vi "Stop Core.vi"(10 "final error code":i32, 11 "DAQ in":refnum<class "DAQ.lvclass">) -> (3 "DAQ out":refnum<class "DAQ.lvclass">)   [LabVIEW 2011, in "DAQ.lvclass"]
doc: "(<B>Filename</B>: Actor Framework.lvlib:Actor.lvclass:Stop Core.vi)\n\nDefines what the actor does before it stops. Use the <B>final error code</B> input to determine whether the actor shut down in response to an error.\n\nBy default, this method does nothing. A descendant class may override it to define behavior, such as shutting down any processes the actor initiated in its override of the Actor Core method."
uses:
  DAQ.lvclass
  <userlib>/_Frameworks/ActorFramework/Actor/Actor.lvclass
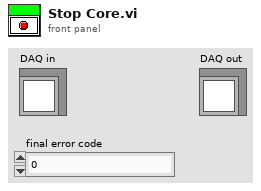
[diagram p1: front panel]
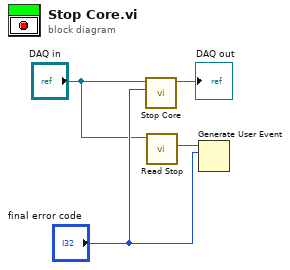
[diagram p0: block diagram]
diagram:
  n1 = call-parent "Stop Core.vi"("final error code"="final error code", "Actor in"="DAQ in") -> ("Actor out"=→"DAQ out":refnum<class "DAQ.lvclass">)  [unwired: 9 in]
  n2 = call "Read Stop.vi"("DAQ in"="DAQ in") -> ("Stop"=w4:refnum<user-event>)  [unwired: 9 in, 1 out]
  n3 = Generate User Event(user event=w4, event data cluster="final error code") -> ()  [unwired: 1 in, 2 out]
